vi "MW Power sweep.vi"() -> ()   [LabVIEW 2012]
uses:
  <vilib>/Analysis/1siggen.llb/Ramp Pattern by Samples.vi
  <vilib>/Utility/file.llb/Write To Spreadsheet File (DBL).vi
  <vilib>/Analysis/NI_AALBase.lvlib
panel:
  in  "Channel":bool=TRUE
  in  "leveling file":path=path "C:/Users/Ouyang Group/Documents/Data/8-26-16/Windfreak plus switches and amp power calibration high res"
  in  "leveling":bool=TRUE
  out "Power":dbl
  out "Freq":dbl
  out "COM Error":bool
  out "Level":bool
  in  "p (dbm)":dbl=-9.0
  in  "file path (dialog if empty)":path
  in  "resolution (1 Hz:1)":i32(ring)=1 items=["0.1 Hz", "1 Hz", "10 Hz", "100 Hz", "1 KHz", "10 KHz", "100 KHz", "1 MHz", "10 MHz", "100 MHz", "1 GHz"]
  in  "band (1-26.5 GHz:20)":i32(ring)=2
  in  "GPIB Address":string="19"
  in  "f start":dbl=1000000000.0 format="%0.2f"
  in  "f end":dbl=4000000000.0 format="%0.2f"
  in  "f samples":i32=50
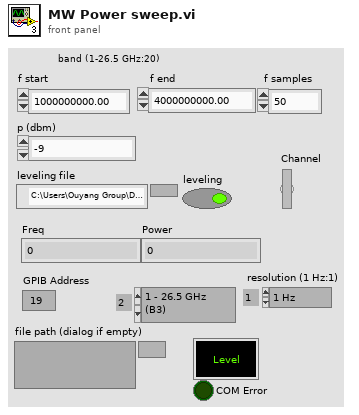
[diagram p1: front panel]
types:
  T1 = cluster{"power\nmeter":bool, bool, "Power Offset":ext}
  T2 = cluster{"source lock":bool, "lock frequency (Hz)":ext, "coarse tune":bool}
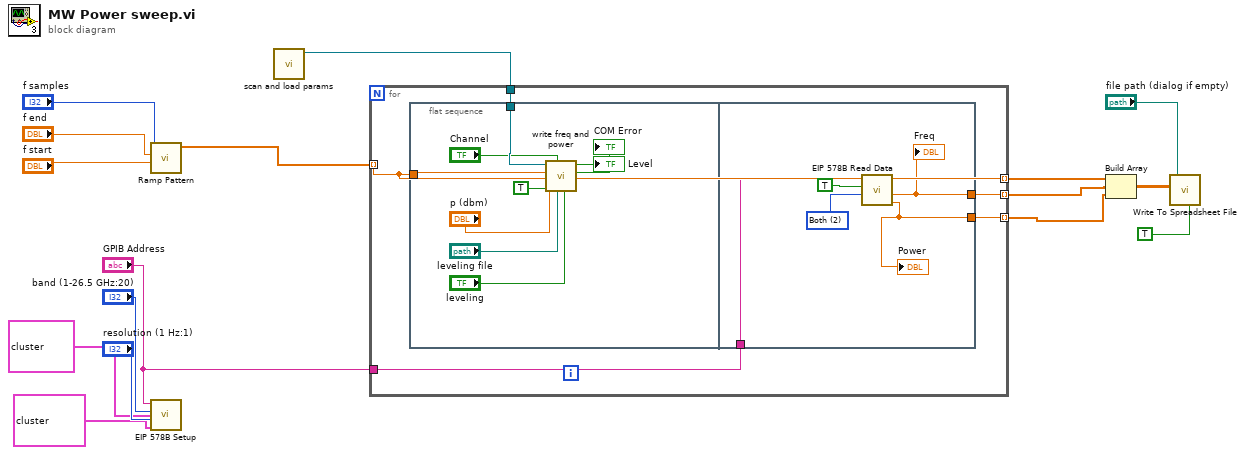
[diagram p0: block diagram]
diagram:
  n1 = call-poly <vilib>:"Ramp Pattern.vi"("start"="f start", "end"="f end", "samples"="f samples") -> ("Ramp Pattern"=w6:dbl[])  [unwired: 7 in, 1 out]
  n2 = call "EIP 578B Setup.vi"("GPIB Address"="GPIB Address", "band (1-26.5 GHz:20)"="band (1-26.5 GHz:20)", "resolution (1 Hz:1)"="resolution (1 Hz:1)", "source locking"=T2 {"source lock"=FALSE, "lock frequency (Hz)"=1000000000.0, "coarse tune"=FALSE}, "power meter"=T1 {"power\nmeter"=TRUE, FALSE, "Power Offset"=0.0}) -> ()  [unwired: 1 in, 2 out]
  n3 = call "scan and load params.vi"() -> ("Serial Port Select"=w1:refnum<visa-resource-name>)  [unwired: 9 out]
  n4 = for {
    tunnel: "GPIB Address" -> [w21]
    tunnel: [w20] -> w5 mode=indexing
    tunnel: w6 -> [w18] mode=indexing
    tunnel: [w19] -> w3 mode=indexing
    tunnel: [w18] -> w2 mode=indexing
    tunnel: w1 -> [w17]
    n5 = flat-sequence {
      tunnel: w18 -> [w26]
      tunnel: w17 -> [w30]
      tunnel: w21 -> [w33]
      tunnel: [w31] -> w20
      tunnel: [w32] -> w19
      frame #0 {
        n6 = call "write freq and power.vi"("leveling"="leveling", "leviling file"="leveling file", "Channel"="Channel", "RF On"=TRUE, "p (dbm)"="p (dbm)", "f (Hz)"=w26, "Serial Port Select"=w30) -> ("COM Error"=→"COM Error":bool, "Level"=→"Level":bool)  [unwired: 3 in]
      }
      frame #1 {
        w35 = 2 items=["Frequency", "Power", "Both"] ("output mode (freq:0)")
        n7 = call "EIP 578B Read Data.vi"("output mode (freq:0)"=w35, "fast (T=active)"=TRUE, "GPIB"=w33) -> ("Power (dBm)"=w32:ext, "frequency (Hz)"=w31:ext)  [unwired: 1 in, 2 out]
        "Power" <- w32
        "Freq" <- w31
      }
    }
  }
  n8 = Build Array(w2, w5, w3) -> (w4:ext[][])
  n9 = call-poly <vilib>:"Write To Spreadsheet File.vi"("transpose? (no:F)"=TRUE, "2D data"=w4, "file path (dialog if empty)"="file path (dialog if empty)") -> ()  [unwired: 5 in, 1 out]
